vi "Measurement UI.vi"() -> ()   [LabVIEW 2024, in "NIScopeFrequencyDomain.lvlib"]
uses:
  NIScopeFrequencyDomain.lvlib
panel:
  out "Actual Sample Rate":dbl
  out "Detected Tones":string[][](table)
  out "Voltage Waveform":waveform(dbl)(graph)
  out "Frequency Spectrum":cluster{dbl[], dbl[]}[](graph)
  out "Frequencies (Hz)":dbl[](array[numeric])
  out "Amplitudes (V)":dbl[](array[numeric])
  out "Magnitude Peak":cluster{dbl[], dbl[]}
  out "Magnitude RMS":cluster{dbl[], dbl[]}
  in  "Trigger Level (V)":dbl format="%.2g"
  out "Waveform Data":dbl[](array[numeric])
  in  "Trigger Slope":i32(ring) items=["Positive", "Negative"]
  in  "Trigger Coupling":u32(ring)=1 items=["AC"=0, "DC"=1, "HF Reject"=3, "LF Reject"=4, "AC Plus HF Reject"=1001]
  in  "Minimum Record Length (S)":i32=20000
  in  "Minimum Sample Rate (S/s)":dbl=10000.0 format="%#.2p"
  in  "Vertical Coupling":i32(ring)=1 items=["AC", "DC", "Ground"]
  in  "Vertical Offset (V)":dbl format="%.2p"
  in  "Vertical Range (V)":dbl=10.0 caption="Vertical Range" format="%.2f"
  in  "Pin Name":string(combo)
  # "Input"
  # "Output"
  # "Pin Settings"
  # "Timing and Trigger Settings"
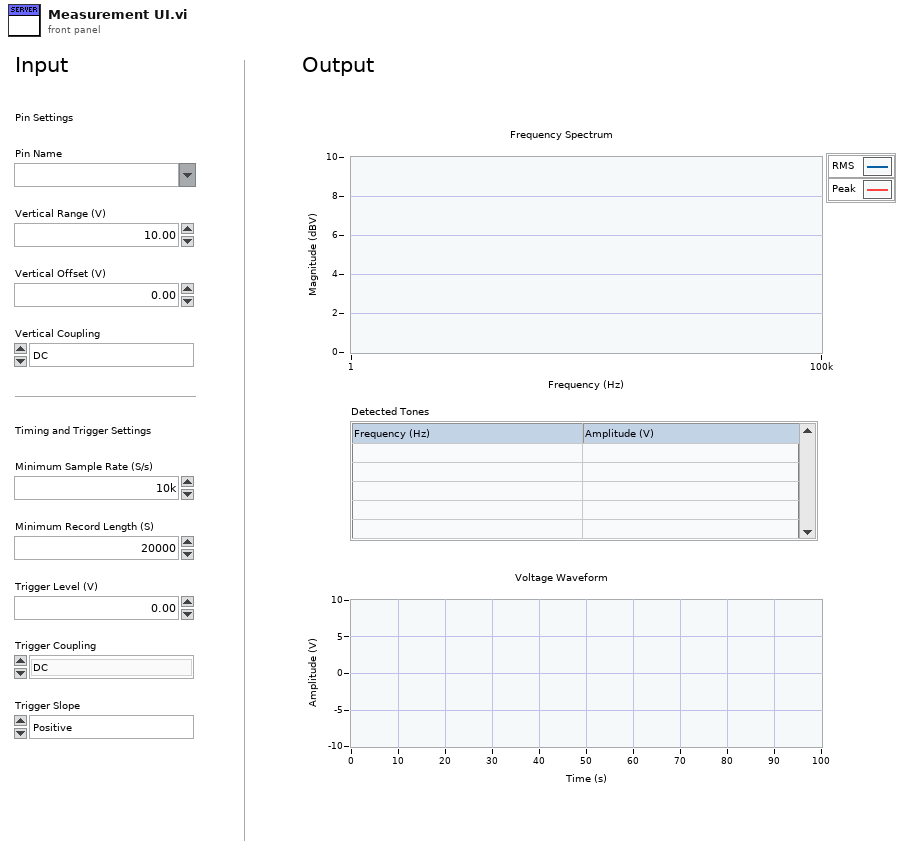
[diagram p1: front panel]
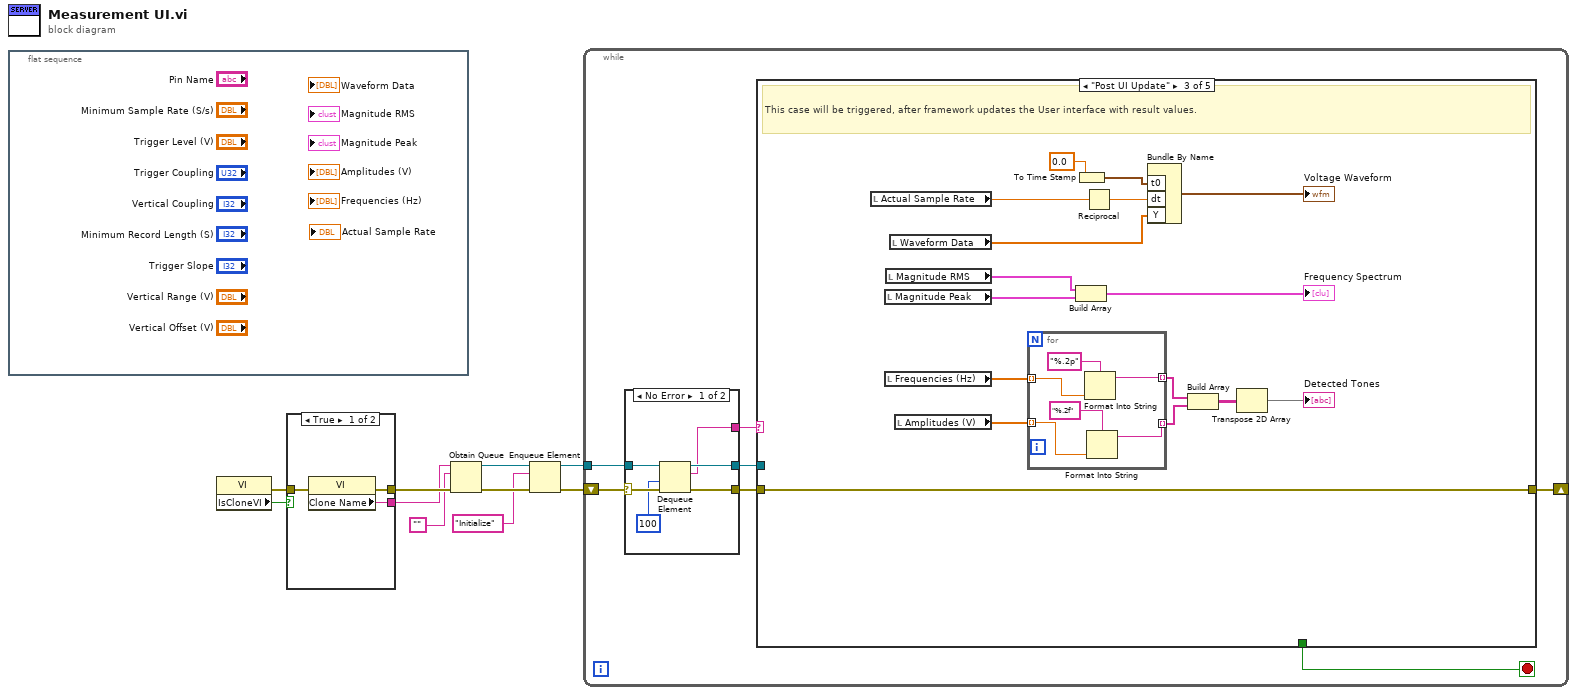
[diagram p0: block diagram]
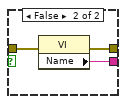
[diagram p2: hidden frame]
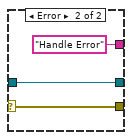
[diagram p3: hidden frame]
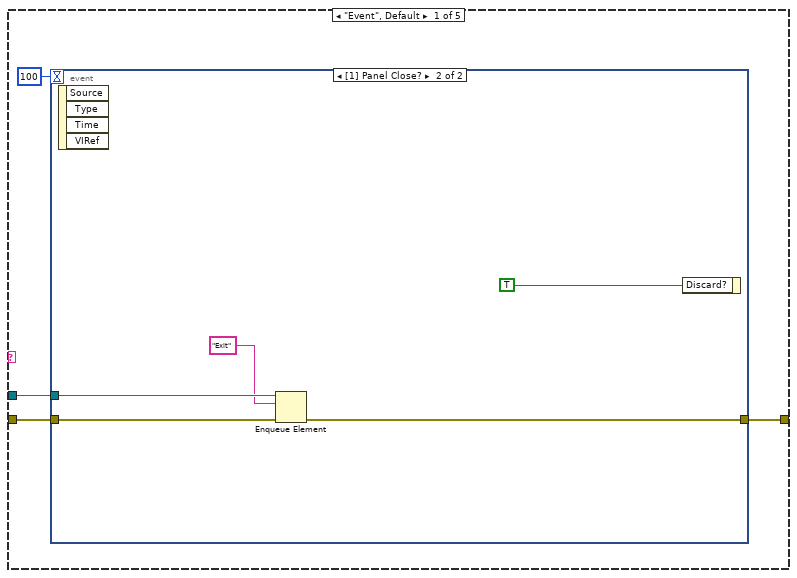
[diagram p4: hidden frame]
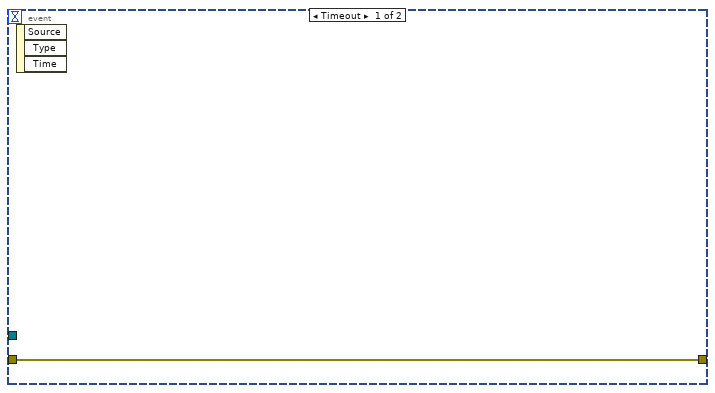
[diagram p5: hidden frame]
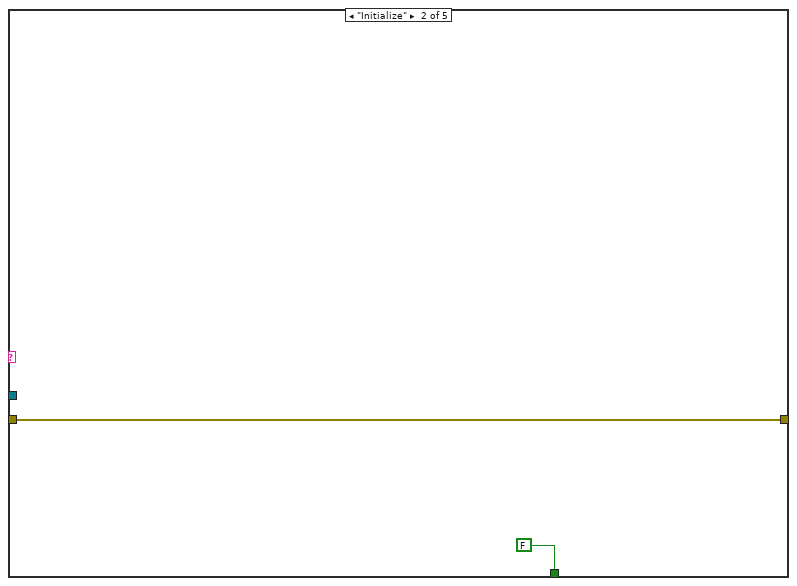
[diagram p6: hidden frame]
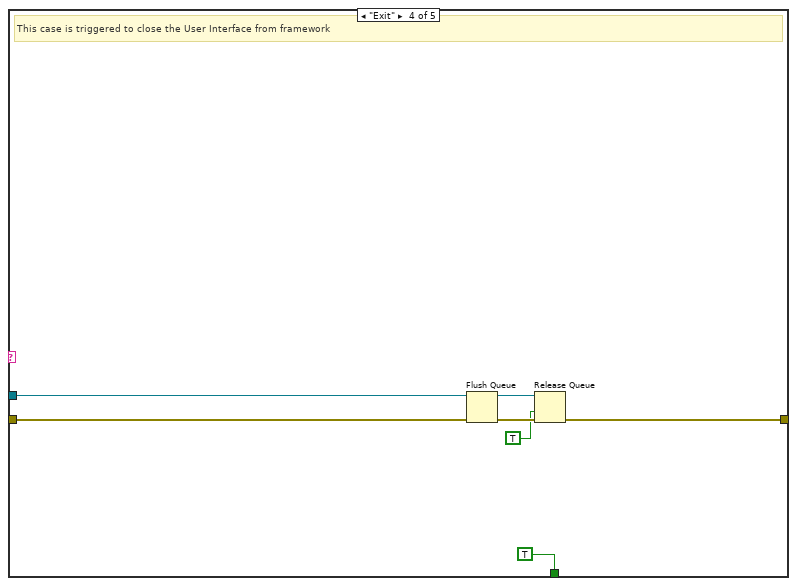
[diagram p7: hidden frame]
diagram:
  n1 = flat-sequence {
    frame #0 {
    }
  }
  n2 = property class="VI"() -> (error out=w1:errorcluster, "IsCloneVI"=w2:bool)  [unwired: 2 in, 1 out]
  n3 = case shown="True" w2 {
    tunnel: [w13 w16] -> w10
    tunnel: [w12 w15] -> w9
    tunnel: w1 -> [w11 w14]
    frame True {
      n4 = property class="VI"(error in=w11) -> (error out=w13:errorcluster, "Clone Name"=w12:string)  [unwired: 1 in, 1 out]
    }
    frame False {
      n5 = property class="VI"(error in=w14) -> (error out=w16:errorcluster, "Name"=w15:string)  [unwired: 1 in, 1 out]
    }
  }
  n6 = Obtain Queue(name (unnamed)=w9, element data type="", error in (no error)=w10) -> (queue out=w6:refnum<queue>, error out=w8:errorcluster)  [unwired: 2 in, 1 out]
  n7 = Enqueue Element(queue=w6, element="Initialize", error in (no error)=w8) -> (queue out=w5:refnum<queue>, error out=w7:errorcluster)  [unwired: 1 in, 1 out]
  n8 = while {
    shift-right: [w18] -> _
    shift-left: w7 -> [w23]
    tunnel: w5 -> [w21]
    stop <- w17 stop-if-true
    n9 = case shown="No Error" w23 {
      selector: w23 -> [w29 w32]
      tunnel: [w28 w32] -> w22
      tunnel: w21 -> [w27 w31]
      tunnel: [w26 w31] -> w20
      tunnel: [w25 "Handle Error"] -> w19
      frame No Error {
        n10 = Dequeue Element(queue=w27, timeout in ms (-1)=100, error in (no error)=w29) -> (queue out=w26:refnum<queue>, element=w25:string, error out=w28:errorcluster)  [unwired: 1 out]
      }
      frame Error {
      }
    }
    n11 = case shown="\"Post UI Update\"" w19 {
      tunnel: w22 -> [w35 w44 w60 w73 w74]
      tunnel: w20 -> [w33 _ _ w71 _]
      tunnel: [w36 w44 w60 w68 w74] -> w18
      tunnel: [_ FALSE _ TRUE _] -> w17
      frame "Event", Default {
        n12 = event shown="[1] Panel Close?" {
          selector: _ -> [_ _]
          dyn-events: _ -> [_ _]
          timeout: 100 -> [_ _]
          tunnel: [w37 w40] -> w36
          tunnel: w35 -> [w37 w41]
          tunnel: w33 -> [_ w39]
          event Timeout {
            n13 = event-data() -> ()  [unwired: 1 in, 3 out]
          }
          event Panel Close? {
            n14 = event-data() -> ()  [unwired: 1 in, 4 out]
            n15 = Enqueue Element(queue=w39, element="Exit", error in (no error)=w41) -> (error out=w40:errorcluster)  [unwired: 1 in, 2 out]
            n16 = event-data("Discard?"=TRUE) -> ()  [unwired: 1 in, 1 out]
          }
        }
      }
      frame "Initialize" {
      }
      frame "Post UI Update" {
        # "This case will be triggered, after framework updates the User interface with result values."
        n17 = local read "Actual Sample Rate"() -> (w51:dbl)
        n18 = local read "Magnitude Peak"() -> (w54:cluster{dbl[], dbl[]})
        n19 = local read "Frequencies (Hz)"() -> (w50:dbl[])
        n20 = local read "Magnitude RMS"() -> (w52:cluster{dbl[], dbl[]})
        n21 = local read "Waveform Data"() -> (w56:dbl[])
        n22 = local read "Amplitudes (V)"() -> (w49:dbl[])
        n23 = for {
          tunnel: w50 -> [w66] mode=indexing
          tunnel: w49 -> [w63] mode=indexing
          tunnel: [w64] -> w48 mode=indexing
          tunnel: [w62] -> w47 mode=indexing
          n24 = Format Into String(format string="%.2p", w66) -> (resulting string=w64:string)  [unwired: 2 in, 1 out]
          n25 = Format Into String(format string="%.2f" ("initial string"), w63) -> (resulting string=w62:string)  [unwired: 2 in, 1 out]
        }
        n26 = Build Array(w52, w54) -> (→"Frequency Spectrum":cluster{dbl[], dbl[]}[])
        n27 = To Time Stamp(1:0.0 ("t0")) -> (0:w58:timestamp)
        n28 = Reciprocal(x=w51) -> (1/x=w57:dbl)
        n29 = Bundle By Name("t0"=w58, "dt"=w57, "Y"=w56) -> (→"Voltage Waveform":waveform(dbl))  [unwired: 1 in]
        n30 = Build Array(w48, w47) -> (w46:string[][])
        n31 = Transpose 2D Array(2D array=w46) -> (transposed array=→"Detected Tones":string[][])
      }
      frame "Exit" {
        # "This case is triggered to close the User Interface from framework"
        n32 = Flush Queue(queue=w71, error in (no error)=w73) -> (queue out=w70:refnum<queue>, error out=w69:errorcluster)  [unwired: 1 out]
        n33 = Release Queue(queue=w70, force destroy? (F)=TRUE, error in (no error)=w69) -> (error out=w68:errorcluster)  [unwired: 2 out]
      }
      frame "Handle Error" {
      }
    }
  }
